vi "GPSDO Controller.vi"() -> ()   [LabVIEW 2015]
uses:
  <vilib>/Instr/_visa.llb/VISA Configure Serial Port (Instr).vi
panel:
  out "CNT No Change Votes":dbl
  out "CNT Down Votes":dbl
  out "CNT Up Votes":dbl
  out "RS No Change Votes":dbl
  out "RS Down Votes":dbl
  out "Running Sum":dbl(graph)
  in  "Clear":bool
  in  "Baud Rate":dbl=115200.0
  in  "COM Port":refnum<visa-resource-name>
  out "Error Out":errorcluster
  in  "Error In":errorcluster
  out "Tracked Satellites":cluster{dbl, dbl}(graph)
  in  "Save DAC to EEPROM":bool
  in  "Reset GPS":bool
  in  "Set DAC":dbl
  in  "Update DAC":bool
  in  "Change Algorithim":bool
  out "UpTime":string
  out "Warmed Up?":bool
  out "Enforce Warmup":bool
  out "Algorithim In Use":string
  out "Antenna Status":string
  out "Time":string
  in  "Stop":bool
  out "Raw Data":string
  out "Date":string
  out "RS Up Votes":dbl
  out "Running Sum":dbl
  out "DAC Value":dbl
  out "Adjustments Made":dbl
  out "Samples":dbl
  out "Error (mHz)":dbl
  out "Count":cluster{dbl, dbl}(graph)
  out "Longitude":dbl format="%#_9g"
  out "Latitude":dbl
  out "Tracked Satellites":dbl
  out "Visible Satellites":dbl
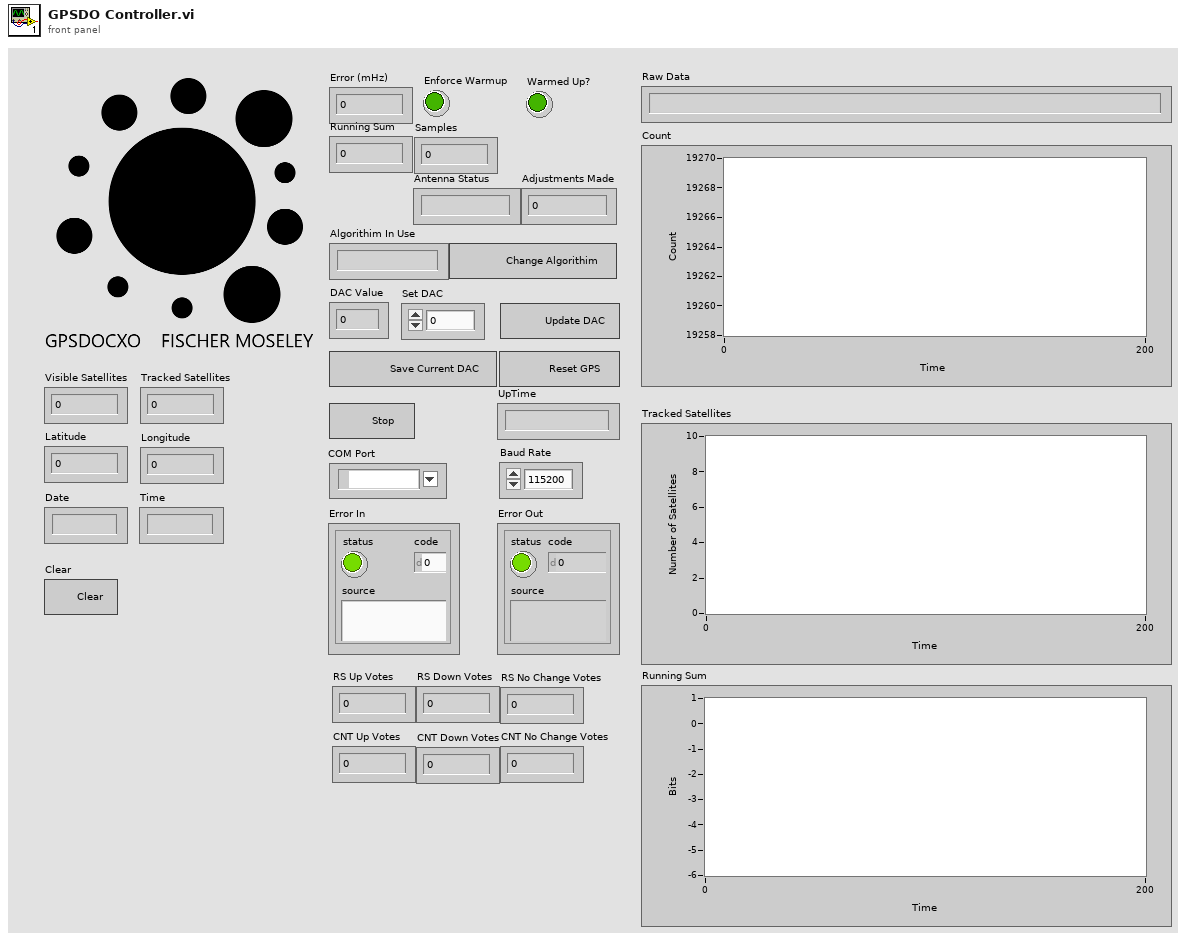
[diagram p1: front panel]
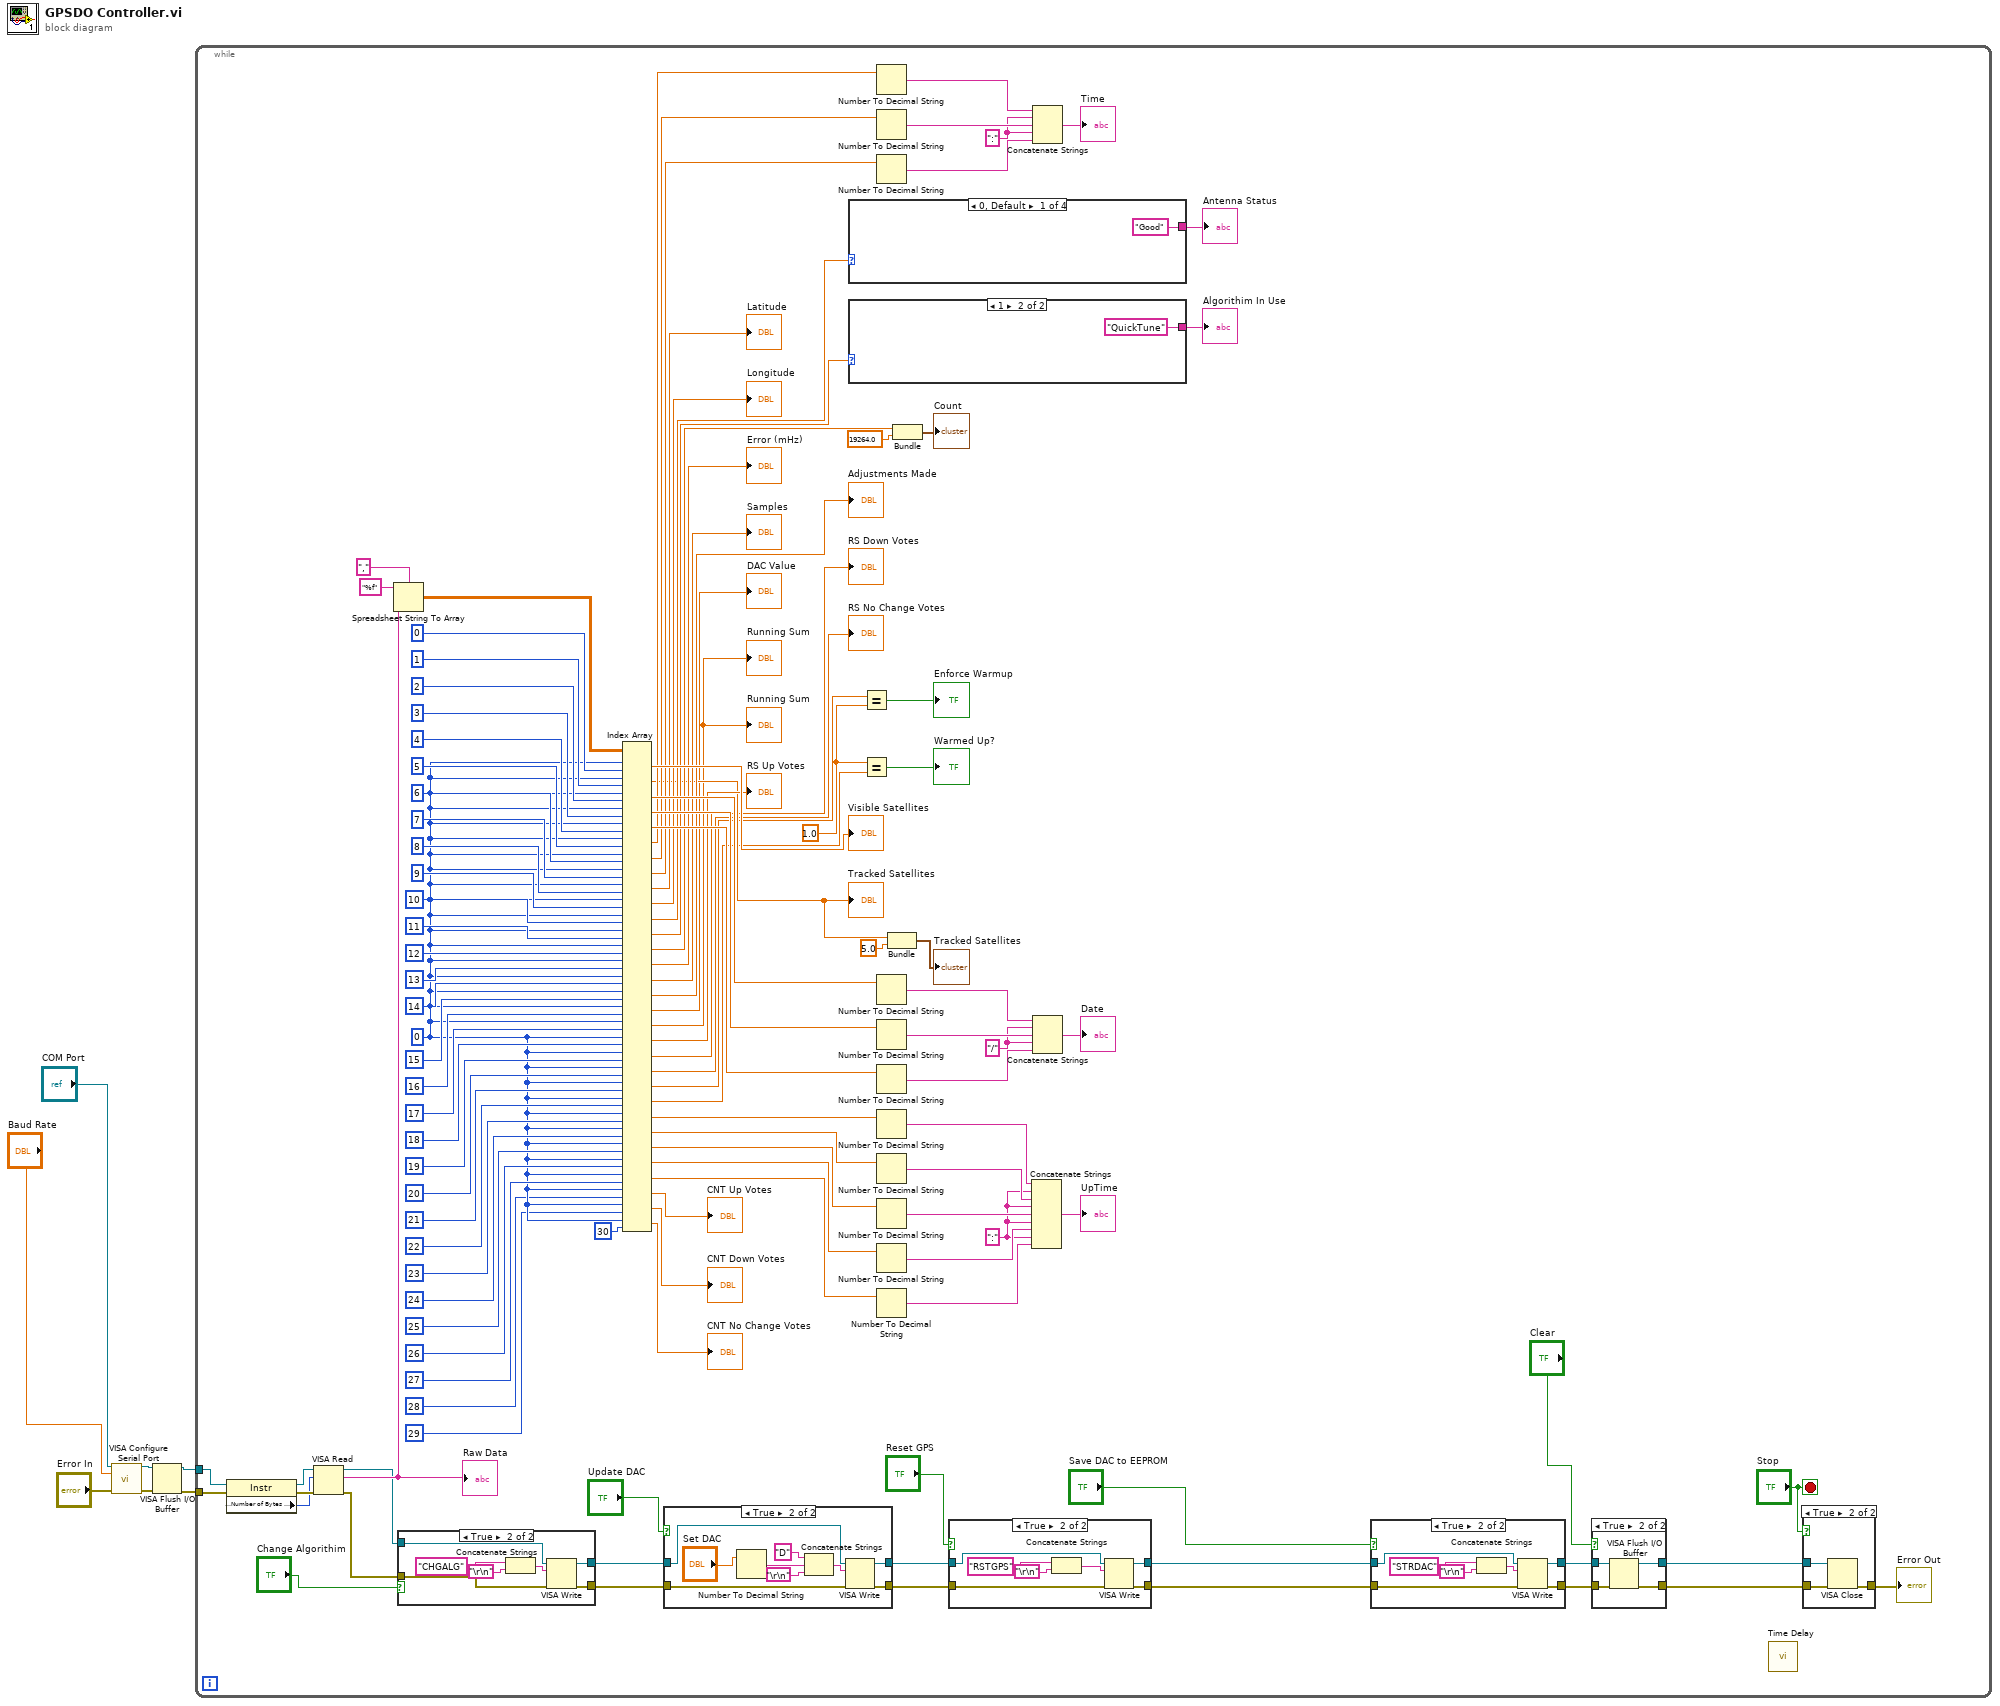
[diagram p0: block diagram]
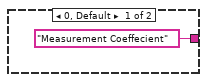
[diagram p7: hidden frame]
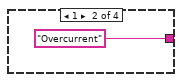
[diagram p8: hidden frame]
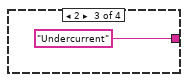
[diagram p9: hidden frame]
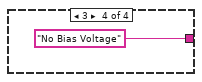
[diagram p10: hidden frame]
diagram:
  n1 = call-poly "VISA Configure Serial Port"("VISA resource name"="COM Port", "baud rate (9600)"="Baud Rate", "error in (no error)"="Error In") -> ("VISA resource name out"=w6:refnum<visa-resource-name>, "error out"=w7:errorcluster)  [unwired: 11 in]
  n2 = VISA Flush I/O Buffer(VISA resource name=w6, error in (no error)=w7) -> (VISA resource name out=w4:refnum<visa-resource-name>, error out=w5:errorcluster)  [unwired: 1 in]
  n3 = while {
    tunnel: w5 -> [w119]
    tunnel: w4 -> [w118]
    stop <- "Stop" stop-if-true
    w63 = ":" ("string")
    w72 = "/" ("string")
    w14 = 0 ("index (row)")
    w106 = ":" ("string")
    w113 = 1.0 ("y")
    n4 = property class="Instr"(reference=w118, error in=w119) -> (reference out=w120:refnum<visa-resource-name>, error out=w122:errorcluster, "Serial Settings:Number of Bytes at Serial Port"=w121:u32)
    n5 = VISA Read(VISA resource name=w120, byte count=w121, error in (no error)=w122) -> (VISA resource name out=w50:refnum<visa-resource-name>, read buffer=w105:string, error out=w51:errorcluster)  [unwired: 1 out]
    "Raw Data" <- w105
    n6 = Spreadsheet String To Array(delimiter (Tab)=",", format string="%f", spreadsheet string=w105) -> (array=w61:dbl[][])  [unwired: 1 in]
    n7 = case shown="True" "Change Algorithim" {
      tunnel: [w161 w168] -> w48
      tunnel: [w160 w167] -> w47
      tunnel: w51 -> [w160 w166]
      tunnel: w50 -> [w161 w165]
      frame False {
      }
      frame True {
        n8 = Concatenate Strings("CHGALG" ("write buffer"), "\r\n") -> (w163:string)
        n9 = VISA Write(VISA resource name=w165, write buffer=w163, error in (no error)=w166) -> (VISA resource name out=w168:refnum<visa-resource-name>, error out=w167:errorcluster)  [unwired: 1 out]
      }
    }
    n10 = Index Array(array=w61, index (row) #1=w14, index (col) #1=0 ("disabled index (col)"), index (row) #2=w14, index (col) #2=1 ("disabled index (col)"), index (row) #3=w14, index (col) #3=2 ("disabled index (col)"), index (row) #4=w14, index (col) #4=3 ("disabled index (col)"), index (row) #5=w14, index (col) #5=4 ("disabled index (col)"), index (row) #6=w14, index (col) #6=5 ("disabled index (col)"), index (row) #7=w14, index (col) #7=6 ("disabled index (col)"), index (row) #8=w14, index (col) #8=7 ("disabled index (col)"), index (row) #9=w14, index (col) #9=8 ("index (col)"), index (row) #10=w14, index (col) #10=9 ("index (col)"), index (row) #11=w14, index (col) #11=10 ("index (col)"), index (row) #12=w14, index (col) #12=11 ("index (col)"), index (row) #13=w14, index (col) #13=12 ("index (col)"), index (row) #14=w14, index (col) #14=13 ("index (col)"), index (row) #15=w14, index (col) #15=14 ("index (col)"), index (row) #16=w14, index (col) #16=15 ("index (col)"), index (row) #17=w14, index (col) #17=16 ("index (col)"), index (row) #18=w14, index (col) #18=17 ("index (col)"), index (row) #19=w14, index (col) #19=18 ("index (col)"), index (row) #20=w14, index (col) #20=19 ("index (col)"), index (row) #21=w14, index (col) #21=20 ("index (col)"), index (row) #22=w14, index (col) #22=21 ("index (col)"), index (row) #23=w14, index (col) #23=22 ("index (col)"), index (row) #24=w14, index (col) #24=23 ("index (col)"), index (row) #25=w14, index (col) #25=24 ("index (col)"), index (row) #26=w14, index (col) #26=25 ("index (col)"), index (row) #27=w14, index (col) #27=26 ("disabled index (col)"), index (row) #28=w14, index (col) #28=27 ("disabled index (col)"), index (row) #29=w14, index (col) #29=28 ("disabled index (col)"), index (row) #30=w14, index (col) #30=29 ("disabled index (col)"), index (row) #31=w14, index (col) #31=30 ("disabled index (col)")) -> (element #1=→"Visible Satellites":dbl, element #2=w35:dbl, element #3=w77:dbl, element #4=w75:dbl, element #5=w70:dbl, element #6=w69:dbl, element #7=w68:dbl, element #8=w67:dbl, element #9=→"Latitude":dbl, element #10=→"Longitude":dbl, element #11=w58:dbl, element #12=w57:dbl, element #13=w38:dbl, element #14=→"Error (mHz)":dbl, element #15=→"Samples":dbl, element #16=→"Adjustments Made":dbl, element #17=→"DAC Value":dbl, element #18=→"Running Sum" →"Running Sum":dbl, element #19=→"RS Up Votes":dbl, element #20=→"RS Down Votes":dbl, element #21=→"RS No Change Votes":dbl, element #22=w22:dbl, element #23=w21:dbl, element #24=w20:dbl, element #25=w19:dbl, element #26=w18:dbl, element #27=w17:dbl, element #28=w16:dbl, element #29=→"CNT Up Votes":dbl, element #30=→"CNT Down Votes":dbl, element #31=→"CNT No Change Votes":dbl)
    "Tracked Satellites" <- w35
    n11 = case shown="True" "Update DAC" {
      tunnel: [w150 w159] -> w45
      tunnel: [w149 w158] -> w44
      tunnel: w47 -> [w149 w157]
      tunnel: w48 -> [w150 w156]
      frame False {
      }
      frame True {
        n12 = Number To Decimal String(number="Set DAC") -> (decimal integer string=w151:string)  [unwired: 1 in]
        n13 = Concatenate Strings("D" ("write buffer"), w151, "\r\n") -> (w154:string)
        n14 = VISA Write(VISA resource name=w156, write buffer=w154, error in (no error)=w157) -> (VISA resource name out=w159:refnum<visa-resource-name>, error out=w158:errorcluster)  [unwired: 1 out]
      }
    }
    n15 = case shown="0, Default" w58 {
      tunnel: ["Good" ("Antenna Status") "Overcurrent" ("Antenna Status") "Undercurrent" ("Antenna Status") "No Bias Voltage" ("Antenna Status")] -> w117
      frame 0, Default {
      }
      frame 1 {
      }
      frame 2 {
      }
      frame 3 {
      }
    }
    "Antenna Status" <- w117
    n16 = case shown="1" w57 {
      tunnel: ["Measurement Coeffecient" ("Algorithim In Use") "QuickTune" ("Algorithim In Use")] -> w116
      frame 0, Default {
      }
      frame 1 {
      }
    }
    "Algorithim In Use" <- w116
    n17 = Equal?(x=w22, y=w113) -> (x = y?=→"Enforce Warmup":bool)
    n18 = Equal?(x=w113, y=w21) -> (x = y?=→"Warmed Up?":bool)
    n19 = Number To Decimal String(number=w69) -> (decimal integer string=w66:string)  [unwired: 1 in]
    n20 = Number To Decimal String(number=w68) -> (decimal integer string=w65:string)  [unwired: 1 in]
    n21 = Number To Decimal String(number=w67) -> (decimal integer string=w64:string)  [unwired: 1 in]
    n22 = Number To Decimal String(number=w77) -> (decimal integer string=w76:string)  [unwired: 1 in]
    n23 = Number To Decimal String(number=w75) -> (decimal integer string=w74:string)  [unwired: 1 in]
    n24 = Number To Decimal String(number=w70) -> (decimal integer string=w73:string)  [unwired: 1 in]
    n25 = Number To Decimal String(number=w20) -> (decimal integer string=w112:string)  [unwired: 1 in]
    n26 = Number To Decimal String(number=w19) -> (decimal integer string=w111:string)  [unwired: 1 in]
    n27 = Number To Decimal String(number=w18) -> (decimal integer string=w110:string)  [unwired: 1 in]
    n28 = Number To Decimal String(number=w17) -> (decimal integer string=w109:string)  [unwired: 1 in]
    n29 = Number To Decimal String(number=w16) -> (decimal integer string=w108:string)  [unwired: 1 in]
    n30 = Bundle(w35, "element"=5.0) -> (→"Tracked Satellites":cluster{dbl, "element":dbl})  [unwired: 1 in]
    n31 = Bundle(w38, "element"=19264.0) -> (→"Count":cluster{dbl, "element":dbl})  [unwired: 1 in]
    n32 = case shown="True" "Reset GPS" {
      tunnel: [w141 w148] -> w42
      tunnel: [w140 w147] -> w41
      tunnel: w44 -> [w140 w146]
      tunnel: w45 -> [w141 w145]
      frame False {
      }
      frame True {
        n33 = Concatenate Strings("RSTGPS" ("write buffer"), "\r\n") -> (w143:string)
        n34 = VISA Write(VISA resource name=w145, write buffer=w143, error in (no error)=w146) -> (VISA resource name out=w148:refnum<visa-resource-name>, error out=w147:errorcluster)  [unwired: 1 out]
      }
    }
    n35 = Concatenate Strings(w112, w106, w111, w106, w110, w106, w109, w106, w108) -> (→"UpTime":string)
    n36 = Concatenate Strings(w66, w63, w65, w63, w64) -> (→"Time":string)
    n37 = Concatenate Strings(w76, w72, w74, w72, w73) -> (→"Date":string)
    n38 = case shown="True" "Save DAC to EEPROM" {
      tunnel: [w132 w139] -> w32
      tunnel: [w131 w138] -> w31
      tunnel: w41 -> [w131 w137]
      tunnel: w42 -> [w132 w136]
      frame False {
      }
      frame True {
        n39 = Concatenate Strings("STRDAC" ("write buffer"), "\r\n") -> (w134:string)
        n40 = VISA Write(VISA resource name=w136, write buffer=w134, error in (no error)=w137) -> (VISA resource name out=w139:refnum<visa-resource-name>, error out=w138:errorcluster)  [unwired: 1 out]
      }
    }
    n41 = case shown="True" "Clear" {
      tunnel: [w126 w128] -> w30
      tunnel: [w125 w127] -> w29
      tunnel: w31 -> [w125 w130]
      tunnel: w32 -> [w126 w129]
      frame False {
      }
      frame True {
        n42 = VISA Flush I/O Buffer(VISA resource name=w129, error in (no error)=w130) -> (VISA resource name out=w128:refnum<visa-resource-name>, error out=w127:errorcluster)  [unwired: 1 in]
      }
    }
    n43 = call "Time Delay"() -> ()  [unwired: 11 in, 1 out]
    n44 = case shown="True" "Stop" {
      tunnel: w30 -> [_ w178]
      tunnel: w29 -> [w175 w176]
      tunnel: [w175 w177] -> w33
      frame False {
      }
      frame True {
        n45 = VISA Close(VISA resource name=w178, error in (no error)=w176) -> (error out=w177:errorcluster)
      }
    }
    "Error Out" <- w33
  }
